vi "Find LabVIEW Dependency String.vi"(7 "64-bit?":bool, 8 "Error In":errorcluster, 10 "LabVIEW Version (2014)":u16=2014) -> (0 "Error Out":errorcluster, 2 "Dependency String":string)   [LabVIEW 2014]
uses:
  <vilib>/Utility/config.llb/Read Key (String).vi
  <vilib>/Utility/config.llb/NI_LVConfig.lvlib
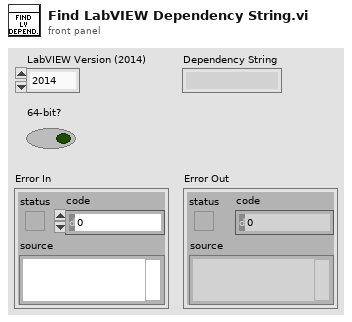
[diagram p1: front panel]
types:
  T1 = typedef "NI_LVConfig.lvlib/Config Data RefNum.ctl" = refnum<k1>
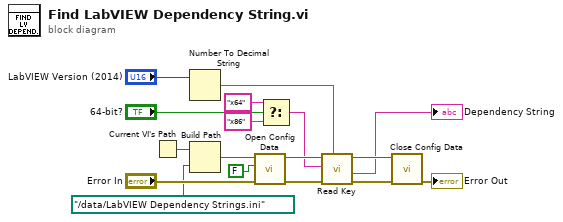
[diagram p0: block diagram]
diagram:
  n1 = Current VI's Path() -> (path=w6:path)
  n2 = Number To Decimal String(number="LabVIEW Version (2014)") -> (decimal integer string=w12:string)  [unwired: 1 in]
  n3 = Build Path(base path=w6, name or relative path=path "../data/LabVIEW Dependency Strings.ini" ("path")) -> (appended path=w5:path)
  n4 = call <vilib>:"Open Config Data.vi"("error in (no error)"="Error In", "create file if necessary (T)"=FALSE, "configuration file path"=w5) -> ("error out"=w4:errorcluster, "refnum"=w16:T1)  [unwired: 6 in, 1 out]
  n5 = Select(t="x64", s="64-bit?", f="x86") -> (s? t:f=w8:string)
  n6 = call-poly <vilib>:"Read Key.vi"("section"=w12, "error in (no error)"=w4, "key"=w8, "refnum"=w16) -> ("error out"=w3:errorcluster, "value"=→"Dependency String":string, "refnum out"=w14:T1)  [unwired: 4 in, 1 out]
  n7 = call <vilib>:"Close Config Data.vi"("error in (no error)"=w3, "refnum"=w14) -> ("error out"=→"Error Out":errorcluster)  [unwired: 8 in, 1 out]
